vi "Claudia_Fun.vi"(10 "Files":T1[](array[typedef])) -> ()   [LabVIEW 2022 SP3]
uses:
  Curtin1_Label.ctl
  GraphType.ctl
  Mic/Mic_Global.vi
panel:
  in  "Tab Control":enum32{"Raw files", "Averages"}(tab)
  in  "keep":bool
  in  "Refresh":bool
  in  "Averages":T2(array[cluster])
  out "FRF":cluster{"x0":dbl, "df":dbl, dbl[]}[](graph)
  # "Welcome to Claudia's Plot\n\nThis VI lets you select different groupings of data sets to look for variations across the means and standard deviations."
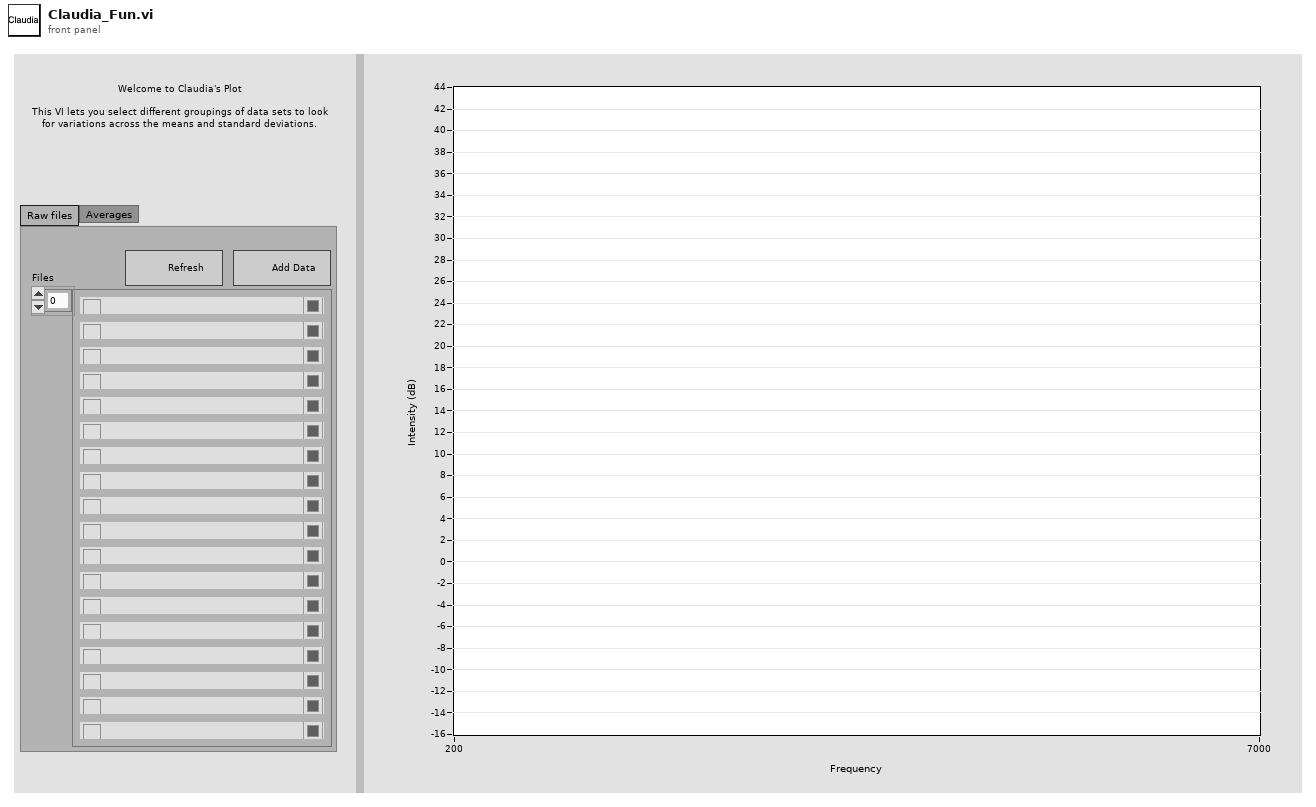
[diagram p1: front panel]
types:
  T1 = typedef "Curtin1_Label.ctl" = cluster{"Show?":bool, "Name":string, "Color":u32, "Path":path, "Show Notes":bool}
  T2 = cluster{"Show?":bool, "Name":string, "Color":u32, "Path":path}[]
  T3 = typedef "GraphType.ctl" = u16
  T4 = cluster{"View Type":u16, "Smoothing":u16, "Bands":u16, "New Band":bool, "rescale Y":bool, "rescale X":bool, "X_Low":dbl, "X_High":dbl, "dB Range":dbl, "Excel":bool, "Y Scaling":bool, "X Scaling":bool, "mag/phase":T3}
  T5 = cluster{"Start freq":dbl, "Hz resolution":dbl, cdb[]}
  T6 = cluster{"Show?":bool, "Name":string, "Color":u32, "Path":path}
  T7 = cluster{"Alerts":bool, "Log X Axis":bool, "dB scale":bool, "Averaging":bool, "Fade":dbl, "Centroids?":bool}
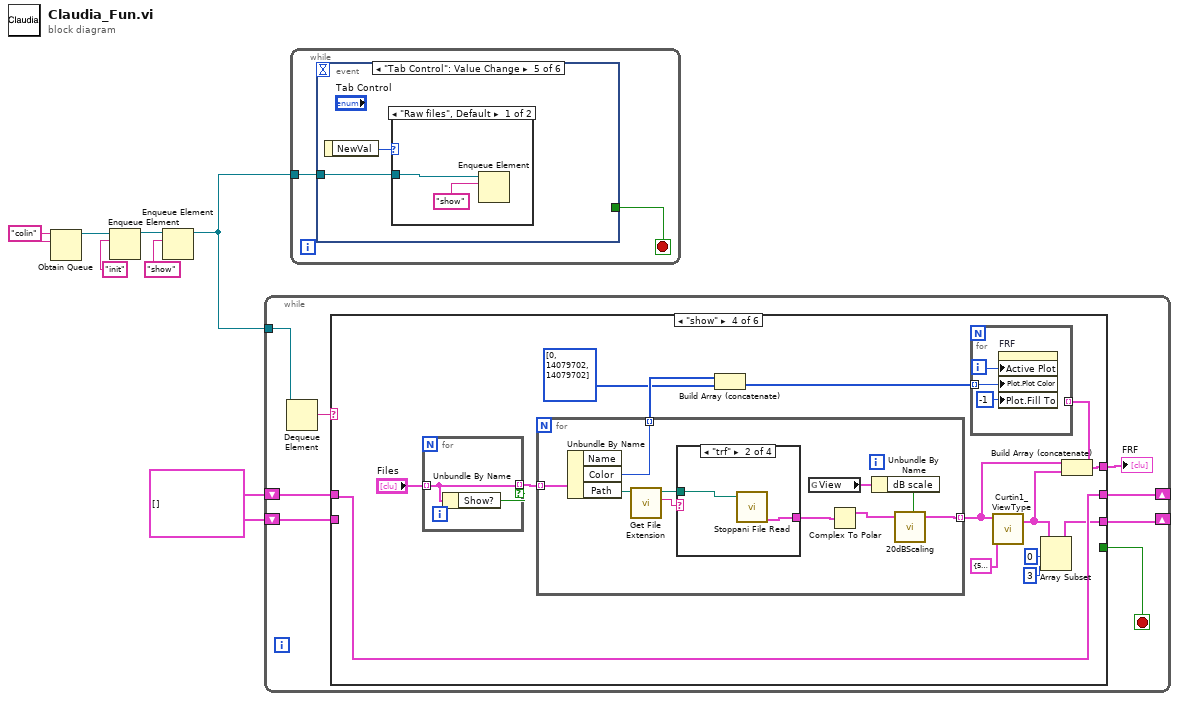
[diagram p0: block diagram]
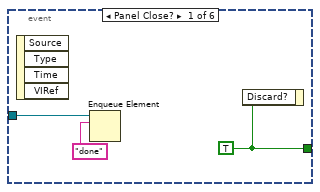
[diagram p2: hidden frame]
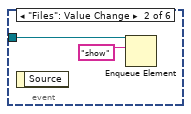
[diagram p3: hidden frame]
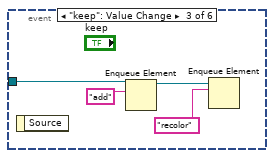
[diagram p4: hidden frame]
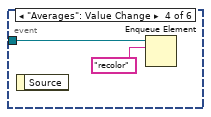
[diagram p5: hidden frame]
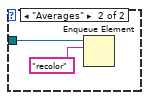
[diagram p6: hidden frame]
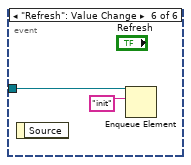
[diagram p7: hidden frame]
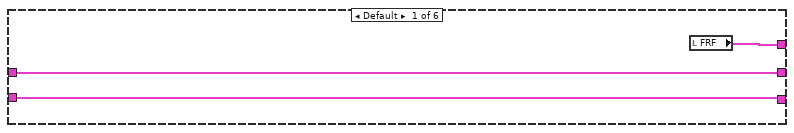
[diagram p8: hidden frame]
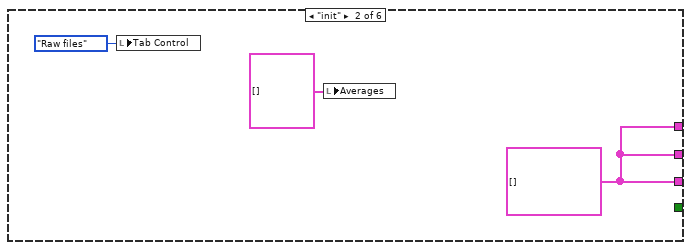
[diagram p9: hidden frame]
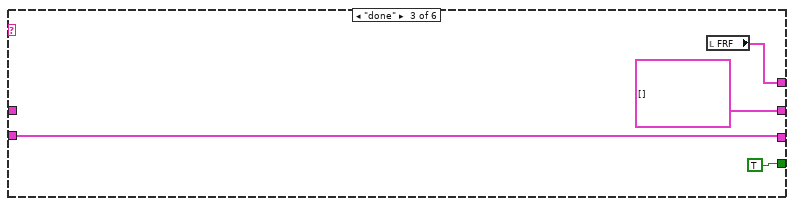
[diagram p10: hidden frame]
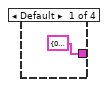
[diagram p11: hidden frame]
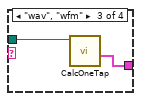
[diagram p12: hidden frame]
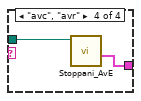
[diagram p13: hidden frame]
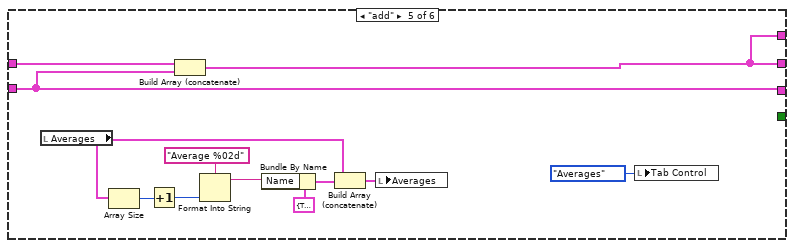
[diagram p14: hidden frame]
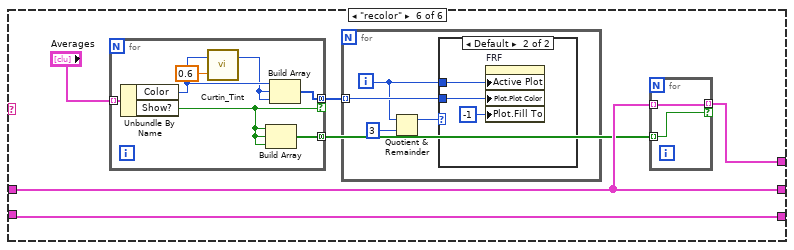
[diagram p15: hidden frame]
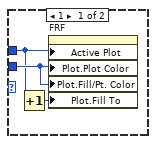
[diagram p16: hidden frame]
diagram:
  w1 = cluster{"x0":dbl, "df":dbl, dbl[]}[] [] ("FRF Out")
  w7 = "colin" ("name (unnamed)")
  n1 = Obtain Queue(name (unnamed)=w7, element data type=w7) -> (queue out=w3:refnum<queue>)  [unwired: 3 in, 2 out]
  n2 = Enqueue Element(queue=w3, element="init") -> (queue out=w2:refnum<queue>)  [unwired: 2 in, 2 out]
  n3 = Enqueue Element(queue=w2, element="show") -> (queue out=w5:refnum<queue>)  [unwired: 2 in, 2 out]
  n4 = while {
    tunnel: w5 -> [w15]
    shift-right: [w12] -> _
    shift-left: w1 -> [w11]
    shift-right: [w8] -> _
    shift-left: w1 -> [w9]
    stop <- w13 stop-if-true
    n5 = Dequeue Element(queue=w15) -> (element=w14:string)  [unwired: 2 in, 3 out]
    n6 = case shown="\"show\"" w14 {
      tunnel: [_ _ TRUE _ _ _] -> w13
      tunnel: [w18 w20 w24 w28 w64 w78] -> w12
      tunnel: w11 -> [w18 _ w24 _ w64 w78]
      tunnel: [w17 w20 w22 w31 w62 w75] -> w10
      tunnel: w9 -> [w16 _ _ w30 w63 w74]
      tunnel: [w16 w20 cluster{"x0":dbl, "df":dbl, dbl[]}[] [] ("FRF Out") w30 w62 w74] -> w8
      frame Default {
        n7 = local read "FRF"() -> (w17:cluster{"x0":dbl, "df":dbl, dbl[]}[])
      }
      frame "init" {
        w20 = cluster{"x0":dbl, "df":dbl, dbl[]}[] [] ("FRF Out")
        n8 = local write "Tab Control"(enum32{"Raw files", "Averages"}."Raw files" ("Tab Control")) -> ()
        n9 = local write "Averages"(T2 [] ("Averages")) -> ()
      }
      frame "done" {
        n10 = local read "FRF"() -> (w22:cluster{"x0":dbl, "df":dbl, dbl[]}[])
      }
      frame "show" {
        n11 = for {
          tunnel: "Files" -> [w42] mode=indexing
          tunnel: [w42] -> w38 mode=indexing if=w43
          n12 = Unbundle By Name(w42) -> ("Show?"=w43:bool)
        }
        n13 = for {
          tunnel: w38 -> [w50] mode=indexing
          tunnel: [w45] -> w35 mode=indexing
          tunnel: [w44] -> w34 mode=indexing
          n14 = Unbundle By Name(w50) -> ("Color"=w44:u32, "Path"=w53:path)  [unwired: 1 out]
          n15 = call <vilib>:"Get File Extension.vi"("file"=w53) -> ("lowercase file extension"=w51:string, "dup file"=w52:path)  [unwired: 6 in, 3 out]
          n16 = case shown="\"trf\"" w51 {
            tunnel: [T5 {"Start freq"=0.0, "Hz resolution"=0.0, []} ("Waveform Graph") w55 w57 w60] -> w49
            tunnel: w52 -> [_ w56 w58 w59]
            frame Default {
            }
            frame "trf" {
              n17 = call "Stoppani File Read.vi"("String in"=w56) -> ("Complex FRF"=w55:cluster{"t0":dbl, "dt":dbl, "Y":cdb[]})  [unwired: 2 in, 3 out]
            }
            frame "wav", "wfm" {
              n18 = call "CalcOneTap.vi"("wavform file"=w58) -> ("Complex FRF"=w57:cluster{dbl, "df":dbl, cdb[]})  [unwired: 7 in, 3 out]
            }
            frame "avc", "avr" {
              n19 = call "Stoppani_AvE.vi"("file (use dialog)"=w59) -> ("Complex FRF"=w60:cluster{"t0":dbl, "df":dbl, "Y":cdb[]})  [unwired: 7 in, 3 out]
            }
          }
          n20 = global read "Mic_Global.vi" "View"() -> (w48:T7)
          n21 = Complex To Polar(r * e^(i*theta)=w49) -> (r=w47:cluster{"t0":dbl, "df":dbl, "Y":dbl[]})  [unwired: 1 out]
          n22 = Unbundle By Name(w48) -> ("dB scale"=w46:bool)
          n23 = call "20dBScaling.vi"("Average FRF in"=w47, "dB?"=w46) -> ("Average FRF out"=w45:cluster{"x0":dbl, "df":dbl, dbl[]})  [unwired: 4 in, 1 out]
        }
        n24 = Build Array (concatenate)(w34, u32[] [0, 14079702, 14079702]) -> (w32:u32[])
        n25 = call "Curtin1_ViewType.vi"("Settings"=T4 {"View Type"=5, "Smoothing"=0, "Bands"=0, "New Band"=FALSE, "rescale Y"=FALSE, "rescale X"=FALSE, "X_Low"=0.0, "X_High"=0.0, "dB Range"=0.0, "Excel"=FALSE, "Y Scaling"=FALSE, "X Scaling"=FALSE, "mag/phase"=0}, "FRF in"=w35) -> ("FRF Out"=w29:cluster{"x0":dbl, "df":dbl, dbl[]}[])  [unwired: 8 in, 1 out]
        n26 = Array Subset(array=w29, index=0, length=3) -> (w28:cluster{"x0":dbl, "df":dbl, dbl[]}[])
        n27 = Build Array (concatenate)(w35, w29) -> (w31:cluster{"x0":dbl, "df":dbl, dbl[]}[])
        n28 = for {
          tunnel: w32 -> [w40] mode=indexing
          tunnel: w31 -> [_] mode=indexing
          i -> [w41]
          n29 = property on="FRF" class="WFGraph (strict)"("Active Plot"=w41, "Plot.Plot Color"=w40, "Plot.Fill To"=i16 -1) -> ()  [unwired: 2 in, 2 out]
        }
      }
      frame "add" {
        n30 = local read "Averages"() -> (w72:T2)
        n31 = Array Size(array=w72) -> (size(s)=w71:i32)
        n32 = Increment(x=w71) -> (x+1=w68:i32)
        n33 = Build Array (concatenate)(w63, w64) -> (w62:cluster{"x0":dbl, "df":dbl, dbl[]}[])
        n34 = Format Into String(format string="Average %02d", w68) -> (resulting string=w66:string)  [unwired: 2 in, 1 out]
        n35 = Bundle By Name(cluster=T6 {"Show?"=TRUE, "Name"="Copy", "Color"=16756736, "Path"=path ""} ("Cluster"), "Name"=w66) -> (w69:T6)
        n36 = Build Array (concatenate)(w72, w69) -> (w61:T2)
        n37 = local write "Averages"(w61) -> ()
        n38 = local write "Tab Control"(enum32{"Raw files", "Averages"}."Averages" ("Tab Control")) -> ()
      }
      frame "recolor" {
        n39 = for {
          tunnel: "Averages" -> [w97] mode=indexing
          tunnel: [w96] -> w76 mode=concatenating if=w95
          tunnel: [w94] -> w73 mode=concatenating
          n40 = Unbundle By Name(w97) -> ("Color"=w93:u32, "Show?"=w95:bool)
          n41 = call "Curtin_Tint.vi"("Tint Factor"=0.6, "Plot.Plot Color"=w93) -> ("Plot.Plot Color 2"=w92:u32)  [unwired: 1 in]
          n42 = Build Array(w95, w95, w95) -> (w94:bool[])
          n43 = Build Array(w93, w92, w92) -> (w96:u32[])
        }
        n44 = for {
          tunnel: w76 -> [w84] mode=indexing
          i -> [w83]
          n45 = Quotient & Remainder(x=w83, y=3) -> (x-y*floor(x/y)=w81:i32)  [unwired: 1 out]
          n46 = case shown="Default" w81 {
            tunnel: w83 -> [w86 w90]
            tunnel: w84 -> [w87 w89]
            frame 1 {
              n47 = Increment(x=w86) -> (x+1=w85:i32)
              n48 = property on="FRF" class="WFGraph (strict)"("Active Plot"=w86, "Plot.Plot Color"=w87, "Plot.Fill/Pt. Color"=w87, "Plot.Fill To"=w85) -> ()  [unwired: 2 in, 2 out]
            }
            frame Default {
              n49 = property on="FRF" class="WFGraph (strict)"("Active Plot"=w90, "Plot.Plot Color"=w89, "Plot.Fill To"=i16 -1) -> ()  [unwired: 2 in, 2 out]
            }
          }
        }
        n50 = for {
          tunnel: [w80] -> w75 mode=indexing if=w79
          tunnel: w74 -> [w80] mode=indexing
          tunnel: w73 -> [w79] mode=indexing
        }
      }
    }
    "FRF" <- w10
  }
  n51 = while {
    tunnel: w5 -> [w98]
    stop <- w99 stop-if-true
    n52 = event shown="[4] \"Tab Control\": Value Change" {
      selector: _ -> [_ _ _ _ _ _]
      dyn-events: _ -> [_ _ _ _ _ _]
      timeout: _ -> [_ _ _ _ _ _]
      tunnel: [w100 _ _ _ _ _] -> w99
      tunnel: w98 -> [w101 w103 w107 w109 w112 w117]
      event Panel Close? {
        w100 = TRUE
        n53 = event-data() -> ()  [unwired: 1 in, 4 out]
        n54 = Enqueue Element(queue=w101, element="done") -> ()  [unwired: 2 in, 3 out]
        n55 = event-data("Discard?"=w100) -> ()  [unwired: 1 in, 1 out]
      }
      event "Files": Value Change {
        n56 = event-data() -> ()  [unwired: 1 in, 1 out]
        n57 = Enqueue Element(queue=w103, element="show") -> ()  [unwired: 2 in, 3 out]
      }
      event "keep": Value Change {
        n58 = event-data() -> ()  [unwired: 1 in, 1 out]
        n59 = Enqueue Element(queue=w107, element="add") -> (queue out=w105:refnum<queue>)  [unwired: 2 in, 2 out]
        n60 = Enqueue Element(queue=w105, element="recolor") -> ()  [unwired: 2 in, 3 out]
      }
      event "Averages": Value Change {
        n61 = event-data() -> ()  [unwired: 1 in, 1 out]
        n62 = Enqueue Element(queue=w109, element="recolor") -> ()  [unwired: 2 in, 3 out]
      }
      event "Tab Control": Value Change {
        n63 = event-data() -> ("NewVal"=w111:enum32{"Raw files", "Averages"})  [unwired: 1 in]
        n64 = case shown="\"Raw files\", Default" w111 {
          tunnel: w112 -> [w113 w115]
          frame "Raw files", Default {
            n65 = Enqueue Element(queue=w113, element="show") -> ()  [unwired: 2 in, 3 out]
          }
          frame "Averages" {
            n66 = Enqueue Element(queue=w115, element="recolor") -> ()  [unwired: 2 in, 3 out]
          }
        }
      }
      event "Refresh": Value Change {
        n67 = event-data() -> ()  [unwired: 1 in, 1 out]
        n68 = Enqueue Element(queue=w117, element="init") -> ()  [unwired: 2 in, 3 out]
      }
    }
  }
